vi "Command Linkages NodeID to GUID.vi"(8 "error in (no error)":errorcluster, 11 "Linked Channels In":T2(array[cluster]) {"Channel Ref in" format="%.0x"}) -> (0 "error out":errorcluster, 3 "Linked Channels out":cluster{"Variable Name":string, "GUID":string}[](array[cluster]))   [LabVIEW 2018, in "Instrument Addon Scripting API.lvlib"]
uses:
  Instrument Addon Scripting API.lvlib
  <vilib>/NI Veristand/Custom Device API/Custom Device Item Ref.ctl
  Addon/Addon Shared/SubVIs/Constants.vi
  <vilib>/NI Veristand/Custom Device API/Get Item Property (String).vi
  <vilib>/NI VeriStand/Custom Device API/Custom Device API.lvlib
  Addon/Addon Shared/Instrument Addon Shared.lvlib
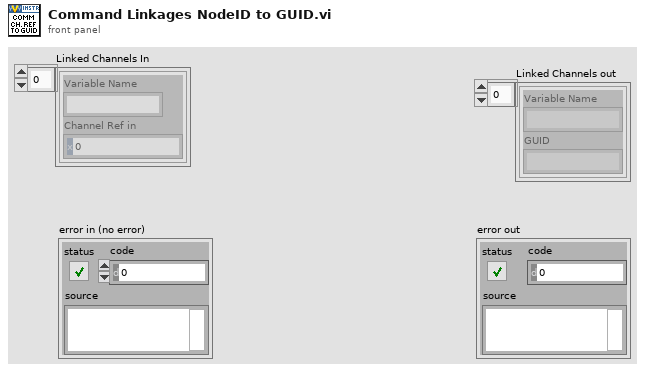
[diagram p1: front panel]
types:
  T1 = typedef "Custom Device API.lvlib/Custom Device Item Ref.ctl" = u64
  T2 = cluster{"Variable Name":string, "Channel Ref in":T1}[]
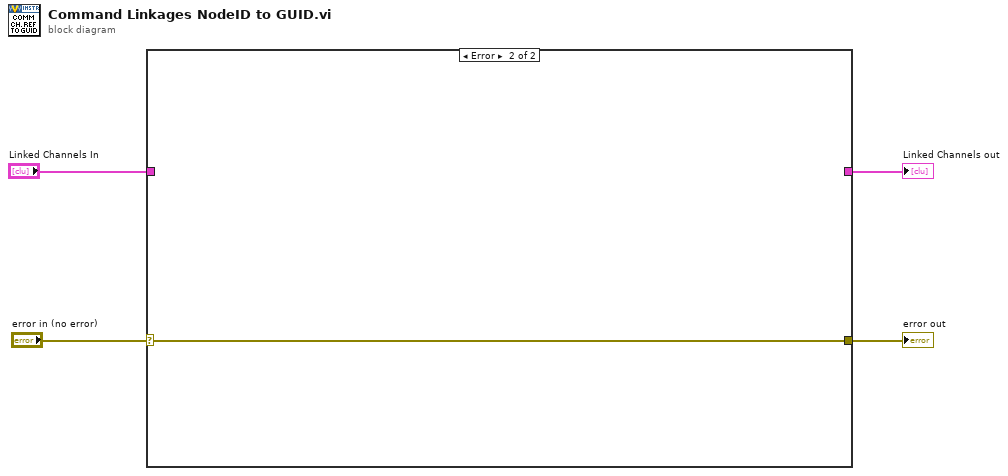
[diagram p0: block diagram]
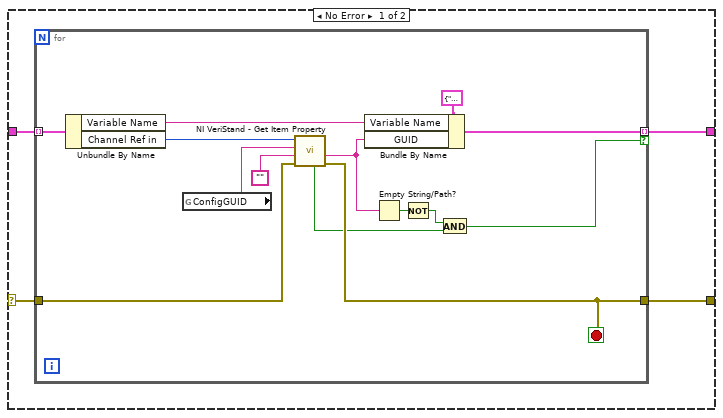
[diagram p2: hidden frame]
diagram:
  n1 = case shown="Error" "error in (no error)" {
    selector: "error in (no error)" -> [w5 w23]
    tunnel: [w8 _] -> w4
    tunnel: [w7 w23] -> w3
    tunnel: "Linked Channels In" -> [w6 _]
    frame No Error {
      n2 = for {
        tunnel: w6 -> [w22] mode=indexing
        tunnel: w5 -> [w17]
        tunnel: [w20] -> w8 mode=indexing if=w19
        tunnel: [w18] -> w7
        stop <- w18 stop-if-true
        n3 = Unbundle By Name(w22) -> ("Variable Name"=w21:string, "Channel Ref in"=w16:T1)
        n4 = global read "Constants.vi" "ConfigGUID"() -> (w15:string)
        n5 = call-poly <vilib>:"NI VeriStand - Get Item Property.vi"("error in (no error)"=w17, "Default Value"="", "Property Name"=w15, "Item Ref in"=w16) -> ("error out"=w18:errorcluster, "Value"=w9:string, "Found?"=w13:bool)  [unwired: 4 in, 1 out]
        n6 = Bundle By Name(cluster=cluster{"Variable Name":string, "GUID":string} {"Variable Name"="", "GUID"=""}, "Variable Name"=w21, "GUID"=w9) -> (w20:cluster{"Variable Name":string, "GUID":string})
        n7 = Empty String/Path?(string/path=w9) -> (empty?=w12:bool)
        n8 = Not(x=w12) -> (.not. x?=w11:bool)
        n9 = And(x=w11, y=w13) -> (x .and. y?=w19:bool)
      }
    }
    frame Error {
    }
  }
  "Linked Channels out" <- w4
  "error out" <- w3
